vi "CALC_MARK_TYPE.vi"(0 "VISA IN":refnum<visa-resource-name>, 1 "Marker number":i32, 2 "Type":string, 5 "error in":errorcluster, 7 "Channel":i32) -> (14 "VISA Out":refnum<visa-resource-name>, 19 "error out":errorcluster)   [LabVIEW 2018, in "PNA-X.lvlib"]
doc: "CALCulate<cnum>:MARKer<mkr>:TYPE <char> \n(Read-Write) Sets the type of the specified marker. \nSee Critical Note \nParameters \n<cnum> Channel number of the measurement. There must be a selected measurement \non that channel. If unspecified, <cnum> is set to 1. \n<mkr> Any marker number from 1 to 10; if unspecified, value is set to 1 \n<char> Choose from: \nNORMal - a marker that stays on the assigned X-axis position unless moved or \nsearching. \nFIXed - a marker that will not leave the assigned X or current Y-axis position. \nExamples CALC:MARK:TYPE NORM \ncalculate2:marker2:type fixed \nQuery Syntax CALCulate<cnum>:MARKer<mkr>:TYPE? \nReturn Type Character \n1540\n\nDefault NORMal"
uses:
  PNA-X.lvlib
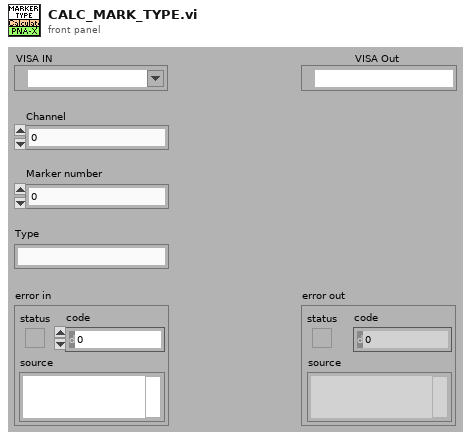
[diagram p1: front panel]
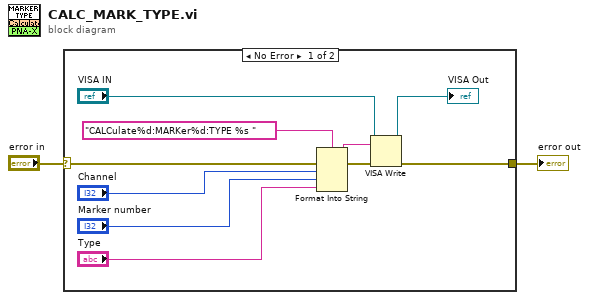
[diagram p0: block diagram]
diagram:
  n1 = case shown="No Error" "error in" {
    selector: "error in" -> [w12 w13]
    tunnel: [w7 w13] -> w1
    frame No Error {
      n2 = Format Into String(format string="CALCulate%d:MARKer%d:TYPE %s " ("Cmdline"), error in=w12, "Channel", "Marker number", "Type") -> (resulting string=w10:string, error out=w11:errorcluster)  [unwired: 1 in]
      n3 = VISA Write(VISA resource name="VISA IN", write buffer=w10, error in (no error)=w11) -> (VISA resource name out=→"VISA Out":refnum<visa-resource-name>, error out=w7:errorcluster)  [unwired: 1 out]
    }
    frame Error {
    }
  }
  "error out" <- w1
